vi "Initialize.vi"(8 "error in":errorcluster, 11 "VS Engine Interface":refnum<class "VS Engine Interface.lvclass">) -> (0 "error out":errorcluster, 3 "Plugin out":refnum<class "Plugin.lvclass">)   [LabVIEW 2024, in "FPGA Addon Engine.lvlib" / "Plugin.lvclass"]
uses:
  Plugin.lvclass
  VS Engine Abstraction/VS Engine Interface/VS Engine Interface.lvclass
  Addon Shared/Types/Compiled.Settings.ctl
  Addon Shared/Types/Compiled.RegisterSettings.ctl
  Addon Shared/Types/Scalar Type.ctl
  Addon Shared/Types/Register Information.ctl
  Addon Shared/Types/FPGA Addon Data Type.ctl
  <vilib>/NI VeriStand/Custom Device API/Block Data Reference.ctl
  <vilib>/NI VeriStand/Custom Device API/Data Reference.ctl
  Addon Shared/Types/Compiled.DMASettings.ctl
  Addon Shared/Types/DMA Settings.ctl
  Addon Shared/Types/Delacing Scheme.ctl
  Addon Shared/Types/DMA Acquisition Mode.ctl
  <vilib>/NI VeriStand/Custom Device API/Waveform Data Reference.ctl
  Addon Shared/Types/FPGA Settings.ctl
  <vilib>/NI VeriStand/Custom Device API/Custom Device Target Type.ctl
  Plugin.lvclass/Plugin.ctl
  VS Plugin Inline Async API/VS Plugin Inline Async API/Types/Error Handling Settings.ctl
  Processes/Output DMA Engine.vi
  Processes/Input DMA Engine.vi
  VS Plugin Inline Async API/VS Plugin Inline Async API/VS Plugin Inline Async API.lvclass
  FPGA Addon Engine.lvlib
  Addon Shared/FPGA Addon Shared.lvlib
  <vilib>/NI VeriStand/Custom Device API/Custom Device API.lvlib
  <vilib>/NI VeriStand/Custom Device Waveform API/Multiple Waveforms Write (DBL)/Multiple Waveforms Write (DBL).lvclass
  <vilib>/NI VeriStand/Custom Device Waveform API/Single Waveform Read (DBL)/Single Waveform Read (DBL).lvclass
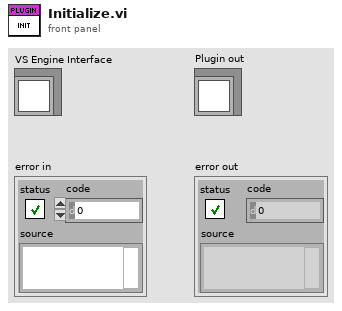
[diagram p1: front panel]
types:
  T1 = typedef "FPGA Addon Shared.lvlib/Compiled.Settings.ctl" = cluster{"Name":string, "IncomingRegisters.Settings":T2[], "IncomingRegisters.Refs":cluster{"Refs":T6[], "Values":dbl[]}, "OutgoingRegisters.Settings":T2[], "OutgoingRegisters.Refs":cluster{"Refs":T6[], "Values":dbl[]}, "Incoming.Size":i32, "Outgoing.Size":i32, "IncomingDMA.Settings":T8[], "OutgoingDMA.Settings":T8[], "FPGA.Settings":T13, "Target.Type":T14}
  T2 = typedef "FPGA Addon Shared.lvlib/Compiled.RegisterSettings.ctl" = cluster{"Scalar Type":T3, "Index":i32, "Length":i32, "Register":T4}
  T3 = typedef "FPGA Addon Shared.lvlib/Scalar Type.ctl" = enum16{"Standard", "Bitpacked"}
  T4 = typedef "FPGA Addon Shared.lvlib/Register Information.ctl" = cluster{"Name":string, "Data Type":T5, "Default Value":variant, "Attributes":variant}
  T5 = typedef "FPGA Addon Shared.lvlib/FPGA Addon Data Type.ctl" = enum8{"<Null>", "I8", "I16", "I32", "I64", "U8", "U16", "U32", "U64", "SGL", "Boolean", "Analog PWM In Settings", "Analog PWM In", "Digital PWM In Settings", "Digital PWM In", "Digital PWM Out", "Sine Out", "FXP", "FXP+/-24.5", "FXP+/-16.5", "FXP+/-32.8", "FXP+/-64.32", "FXP+/-16.7", "FXP+/-20.5", "FXP+/-27.5", "FXP+/-32.16", "FXP+16.3", "FXP+18.3", "Digital Static In", "Digital Static Out", "Digital Static In Settings", "Digital WSS Out", "Quad Encoder Settings", "Quad Encoder In", "Group"}
  T6 = typedef "Custom Device API.lvlib/Block Data Reference.ctl" = cluster{"Data Reference":T7, "Offset":u64, "Length":u64}
  T7 = typedef "Custom Device API.lvlib/Data Reference.ctl" = i32
  T8 = typedef "FPGA Addon Shared.lvlib/Compiled.DMASettings.ctl" = cluster{"Name":string, "Data Type":T5, "DMA.Settings":T9, "DMA.VSRefs":T12[]}
  T9 = typedef "FPGA Addon Shared.lvlib/DMA Settings.ctl" = cluster{"Number of Channels":u8, "Delacing Scheme":T10, "Update Rate":u32, "dt":dbl, "Mode":T11, "Number of Samples":u32, "DMA Host Buffer":u32}
  T10 = typedef "FPGA Addon Shared.lvlib/Delacing Scheme.ctl" = enum8{"Interleaved", "Bitpacked"}
  T11 = typedef "FPGA Addon Shared.lvlib/DMA Acquisition Mode.ctl" = enum8{"Continuous", "Triggered Finite"}
  T12 = typedef "Custom Device API.lvlib/Waveform Data Reference.ctl" = i32
  T13 = typedef "FPGA Addon Shared.lvlib/FPGA Settings.ctl" = cluster{"Bitfile path":path, "RIO Device Address":string, "Group":bool}
  T14 = typedef "Custom Device API.lvlib/Custom Device Target Type.ctl" = enum16{"PharLap", "VxWorks", "Windows", "Linux_32_ARM", "Linux_x64"}
  T15 = typedef "VS Plugin Inline Async API.lvlib/VS Plugin Inline Async API.lvclass/Error Handling Settings.ctl" = cluster{"Write to SystemLog (F)":bool}
  T16 = typedef "FPGA Addon Engine.lvlib/State Variables.ctl" = cluster{"FPGA Ref":refnum<k20>, "IncomingRegisters.Refs":T17[], "IncomingDMA.Refs":T18[], "OutgoingRegisters.Refs":T17[], "OutgoingDMA.Refs":T20[], "Compiled":T1}
  T17 = typedef "FPGA Addon Engine.lvlib/Register Settings.ctl" = cluster{"Name":string, "Data Type":T5, "session":u32, "Scalar Type":T3, "Index":i32, "Length":i32, "attributes":variant, "default value":variant, "RegisterOffset":u32}
  T18 = typedef "FPGA Addon Engine.lvlib/DMA Input References.ctl" = cluster{"Addon Name":string, "Waveform Ref":refnum<class "Multiple Waveforms Write (DBL).lvclass">, "DMA Name":string, "DMA Settings":T9, "Refs":T19}
  T19 = typedef "FPGA Addon Engine.lvlib/DMA Input Refs.ctl" = cluster{"Data Type":T5, "DMA_SGL":refnum<k20>, "DMA_U64":refnum<k20>, "DMA_I64":refnum<k20>, "DMA_FXP+/-32.8":refnum<k20>, "DMA_FXP+/-64.32":refnum<k20>, "DMA_U32":refnum<k20>, "DMA_U16":refnum<k20>, "DMA_U8":refnum<k20>, "DMA_I32":refnum<k20>, "DMA_I16":refnum<k20>, "DMA_I8":refnum<k20>, "DMA_FXP+/-32.16":refnum<k20>}
  T20 = typedef "FPGA Addon Engine.lvlib/DMA Output References.ctl" = cluster{"Addon Name":string, "Waveforms":refnum<class "Single Waveform Read (DBL).lvclass">[], "DMA Name":string, "Refs":T21}
  T21 = typedef "FPGA Addon Engine.lvlib/DMA Output Refs.ctl" = cluster{"Data Type":T5, "DMA_SGL":refnum<k20>, "DMA_U64":refnum<k20>, "DMA_I64":refnum<k20>, "DMA_FXP+/-32.8":refnum<k20>, "DMA_FXP+/-64.32":refnum<k20>, "DMA_U32":refnum<k20>, "DMA_U16":refnum<k20>, "DMA_U8":refnum<k20>, "DMA_I32":refnum<k20>, "DMA_I16":refnum<k20>, "DMA_I8":refnum<k20>, "DMA_FXP+/-32.16":refnum<k20>}
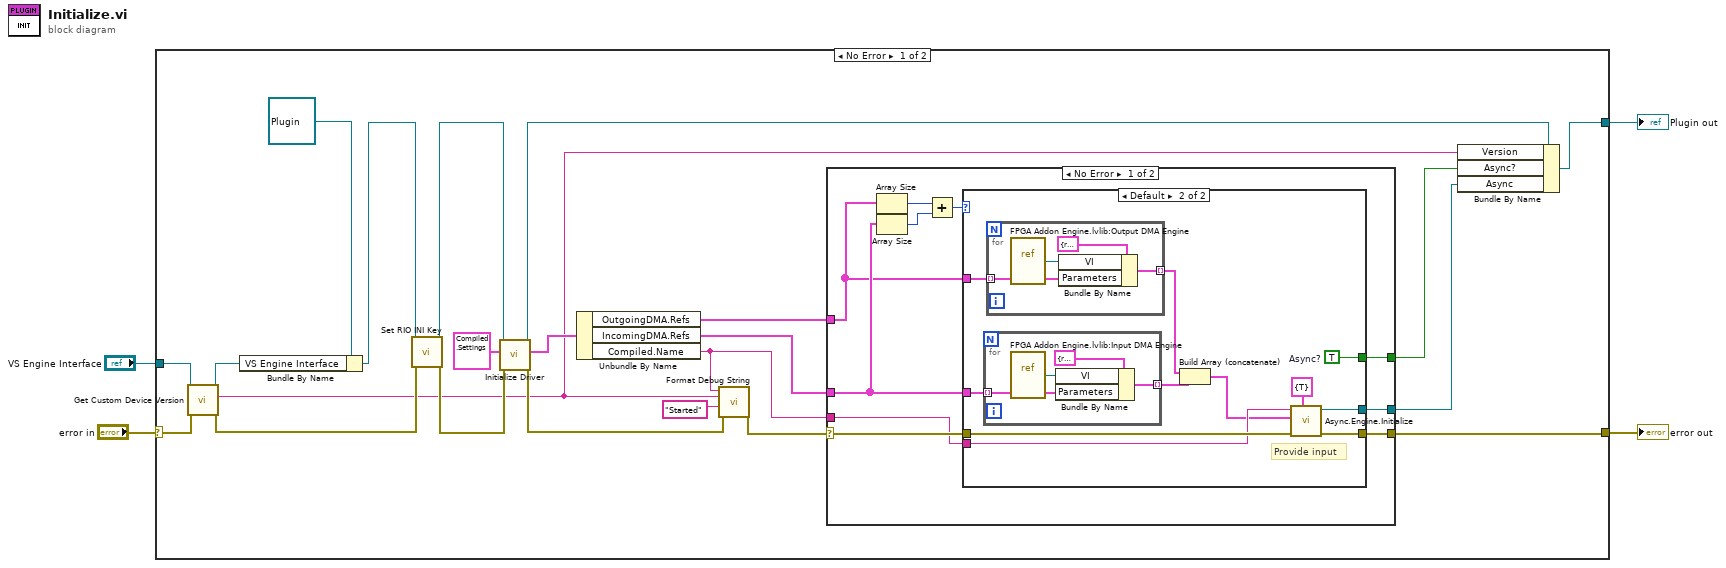
[diagram p0: block diagram]
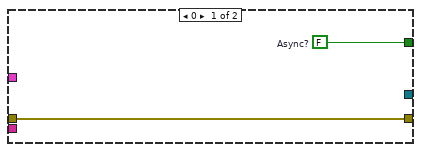
[diagram p2: hidden frame]
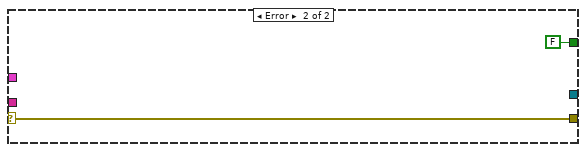
[diagram p3: hidden frame]
diagram:
  n1 = case shown="No Error" "error in" {
    selector: "error in" -> [w22 w60]
    tunnel: [w24 w60] -> w3
    tunnel: [w15 _] -> w2
    tunnel: "VS Engine Interface" -> [w6 _]
    frame No Error {
      n2 = call-dynamic "Get Custom Device Version.vi"("error in"=w22, "VS Engine Interface in"=w6) -> ("error out"=w21:errorcluster, "Version"=w10:string, "VS Engine Interface out"=w5:refnum<class "VS Engine Interface.lvclass">)  [unwired: 7 in]
      n3 = Bundle By Name(cluster=refnum<class "Plugin.lvclass"> refnum ("FPGA Addon Engine.lvlib:Plugin.lvclass"), "VS Engine Interface"=w5) -> (w19:refnum<class "Plugin.lvclass">)
      n4 = call "Set RIO INI Key.vi"("error in"=w21, "Plugin in"=w19) -> ("error out"=w26:errorcluster, "Plugin out"=w18:refnum<class "Plugin.lvclass">)  [unwired: 8 in]
      n5 = call "Initialize Driver.vi"("error in"=w26, "Settings.Compiled"=T1 {"Name"="", "IncomingRegisters.Settings"=[], "IncomingRegisters.Refs"={"Refs"=[], "Values"=[]}, "OutgoingRegisters.Settings"=[], "OutgoingRegisters.Refs"={"Refs"=[], "Values"=[]}, "Incoming.Size"=0, "Outgoing.Size"=0, "IncomingDMA.Settings"=[], "OutgoingDMA.Settings"=[], "FPGA.Settings"={"Bitfile path"=path "", "RIO Device Address"="", "Group"=FALSE}, "Target.Type"=enum."PharLap"}, "Plugin in"=w18) -> ("error out"=w23:errorcluster, "Vars"=w16:T16, "Plugin out"=w9:refnum<class "Plugin.lvclass">)  [unwired: 6 in]
      n6 = Unbundle By Name(w16) -> ("OutgoingDMA.Refs"=w12:T20[], "IncomingDMA.Refs"=w11:T18[], "Compiled.Name"=w8:string)
      n7 = call "Format Debug String.vi"("Version"=w10, "error in (no error)"=w23, "State"="Started" ("string"), "Name"=w8) -> ("error out"=w25:errorcluster)  [unwired: 6 in]
      n8 = case shown="No Error" w25 {
        selector: w25 -> [w35 w59]
        tunnel: [w36 w59] -> w24
        tunnel: [w34 _] -> w13
        tunnel: w11 -> [w33 _]
        tunnel: w12 -> [w32 _]
        tunnel: [w28 FALSE ("Async?")] -> w14
        tunnel: w8 -> [w27 _]
        frame No Error {
          n9 = Array Size(array=w32) -> (size(s)=w31:i32)
          n10 = Array Size(array=w33) -> (size(s)=w30:i32)
          n11 = Add(x=w31, y=w30) -> (x+y=w29:i32)
          n12 = case shown="Default" w29 {
            tunnel: w35 -> [w38 w49]
            tunnel: [w38 w48] -> w36
            tunnel: [_ w44] -> w34
            tunnel: w33 -> [_ w42]
            tunnel: w32 -> [_ w47]
            tunnel: [w37 w45] -> w28
            tunnel: w27 -> [_ w43]
            frame 0 {
              w37 = FALSE  # Async?
            }
            frame Default {
              w45 = TRUE  # Async?
              # "Provide input"
              n13 = for {
                tunnel: w42 -> [w50] mode=indexing
                tunnel: [w52] -> w41 mode=indexing
                n14 = vi-ref "FPGA Addon Engine.lvlib:Input DMA Engine.vi"() -> (w51:refnum<vi>)
                n15 = Bundle By Name(cluster=cluster{"VI":refnum<vi>, "Parameters":variant} {"VI"=refnum, "Parameters"=variant} ("Process"), "VI"=w51, "Parameters"=w50) -> (w52:cluster{"VI":refnum<vi>, "Parameters":variant})
              }
              n16 = for {
                tunnel: w47 -> [w56] mode=indexing
                tunnel: [w55] -> w46 mode=indexing
                n17 = vi-ref "FPGA Addon Engine.lvlib:Output DMA Engine.vi"() -> (w54:refnum<vi>)
                n18 = Bundle By Name(cluster=cluster{"VI":refnum<vi>, "Parameters":variant} {"VI"=refnum, "Parameters"=variant} ("Process"), "VI"=w54, "Parameters"=w56) -> (w55:cluster{"VI":refnum<vi>, "Parameters":variant})
              }
              n19 = Build Array (concatenate)(w46, w41) -> (w40:cluster{"VI":refnum<vi>, "Parameters":variant}[])
              n20 = call "Async.Engine.Initialize.vi"("Error Log Settings"=T15 {"Write to SystemLog (F)"=TRUE}, "error in"=w49, "Processes"=w40, "Name"=w43) -> ("error out"=w48:errorcluster, "VS Plugin Inline Async API out"=w44:refnum<class "VS Plugin Inline Async API.lvclass">)  [unwired: 6 in]
            }
          }
        }
        frame Error {
        }
      }
      n21 = Bundle By Name(cluster=w9, "Version"=w10, "Async?"=w14, "Async"=w13) -> (w15:refnum<class "Plugin.lvclass">)
    }
    frame Error {
    }
  }
  "error out" <- w3
  "Plugin out" <- w2
